vi "Pulse.vi"(0 "Data in":T1, 1 "error in":errorcluster) -> (2 "Data out":T1, 3 "error out":errorcluster, 4 "Ran?":bool)   [LabVIEW 2017, in "Steps.lvlib"]
uses:
  Steps.lvlib
  Type_Defs/Data.ctl
  Type_Defs/Diagnostics.ctl
  Type_Defs/Systems.ctl
panel:
  out "Helical":dbl(graph)
  out "Toroidal":dbl(graph)
  in  "Step Back":bool
  in  "Continue":bool
  # "Verify that the pulse is correct."
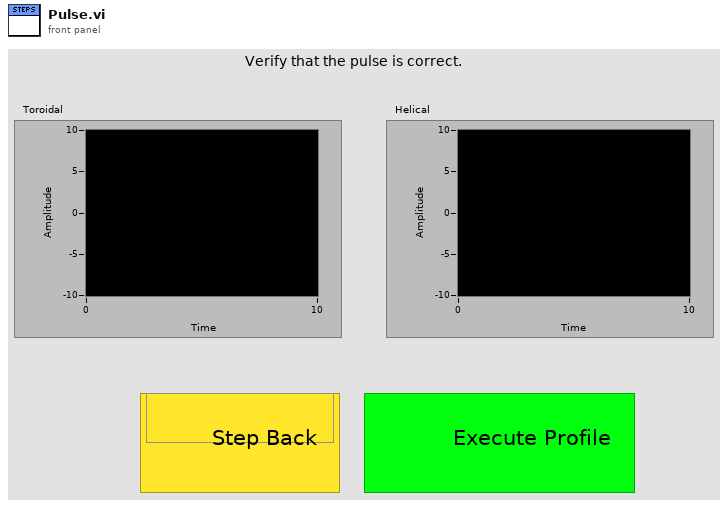
[diagram p1: front panel]
types:
  T1 = typedef "Data.ctl" = cluster{"User Name":string, "Experiment Number":i32, "Start Time":timestamp, "Data":dbl[], "Step Number":i32, "Step Instructions":string, "Diagnostics":T2, "Experiment Purpose":string, "Experiment State":enum16{"Off", "Setting Up", "Ready", "In Progress", "Shutting Down"}, "Systems":T3, "Vacuum Pressure":dbl, "Fieldpoints":cluster{"System Boolean Fieldpoints":cluster{"Compressed Air":refnum<k21>, "T-20kV Power Switch":refnum<k21>, "T-Rectifier":refnum<k21>, "Engage Interlock":refnum<k21>, "Ventilator":refnum<k21>, "Magnetron":refnum<k21>, "H-20kV Power Switch":refnum<k21>, "H-Rectifier":refnum<k21>, "Main Water Pump":refnum<k21>, "WEGA Water Pump":refnum<k21>, "Gas Inlet Valves":refnum<k21>}, "Step Fieldpoints":cluster{"Exhaust Ventillator":refnum<k21>, "Compressed Air":refnum<k21>, "Water Pressure":refnum<k21>, "Interlock":refnum<k21>, "Toroidal Power Supply 1":refnum<k21>, "Toroidal Power Supply 2":refnum<k21>, "Toroidal Rectifier":refnum<k21>, "Helical Power Supply":refnum<k21>, "Helical Rectifier":refnum<k21>, "6kW Magnetron Standby":refnum<k21>, "20kW Magnetron Standby":refnum<k21>}}, "Pressure History":cluster{"Seconds into Experiment":i32[], "Pressure Data":dbl[]}, "Time Computer Control":dbl[], "Toroidal Voltage Computer Control":dbl[], "Helical Voltage Computer Control":dbl[], "Toroidal Current":dbl[], "Toroidal Voltage":dbl[], "Toroidal Current Set Point":dbl[], "Helical Current Set Point":dbl[], "Helical Voltage":dbl[], "Helical Current":dbl[], "Experiment Folder":path, "Run Another Shot?":bool}
  T2 = typedef "Diagnostics.ctl" = cluster{"Langmuir Probe":bool, "Rogowski 1":bool, "Rogowski 2":bool, "Rogowski 3":bool, "B-dot 1":bool, "B-dot 2":bool}
  T3 = typedef "Systems.ctl" = cluster{"Compressed Air":bool, "T-20kV Power Switch":bool, "T-Rectifier":bool, "Engage Interlock":bool, "Ventilator":bool, "Magnetron":bool, "H-20kV Power Switch":bool, "H-Rectifier":bool, "Main Water Pump":bool, "WEGA Water Pump":bool, "Gas Inlet Valves":bool}
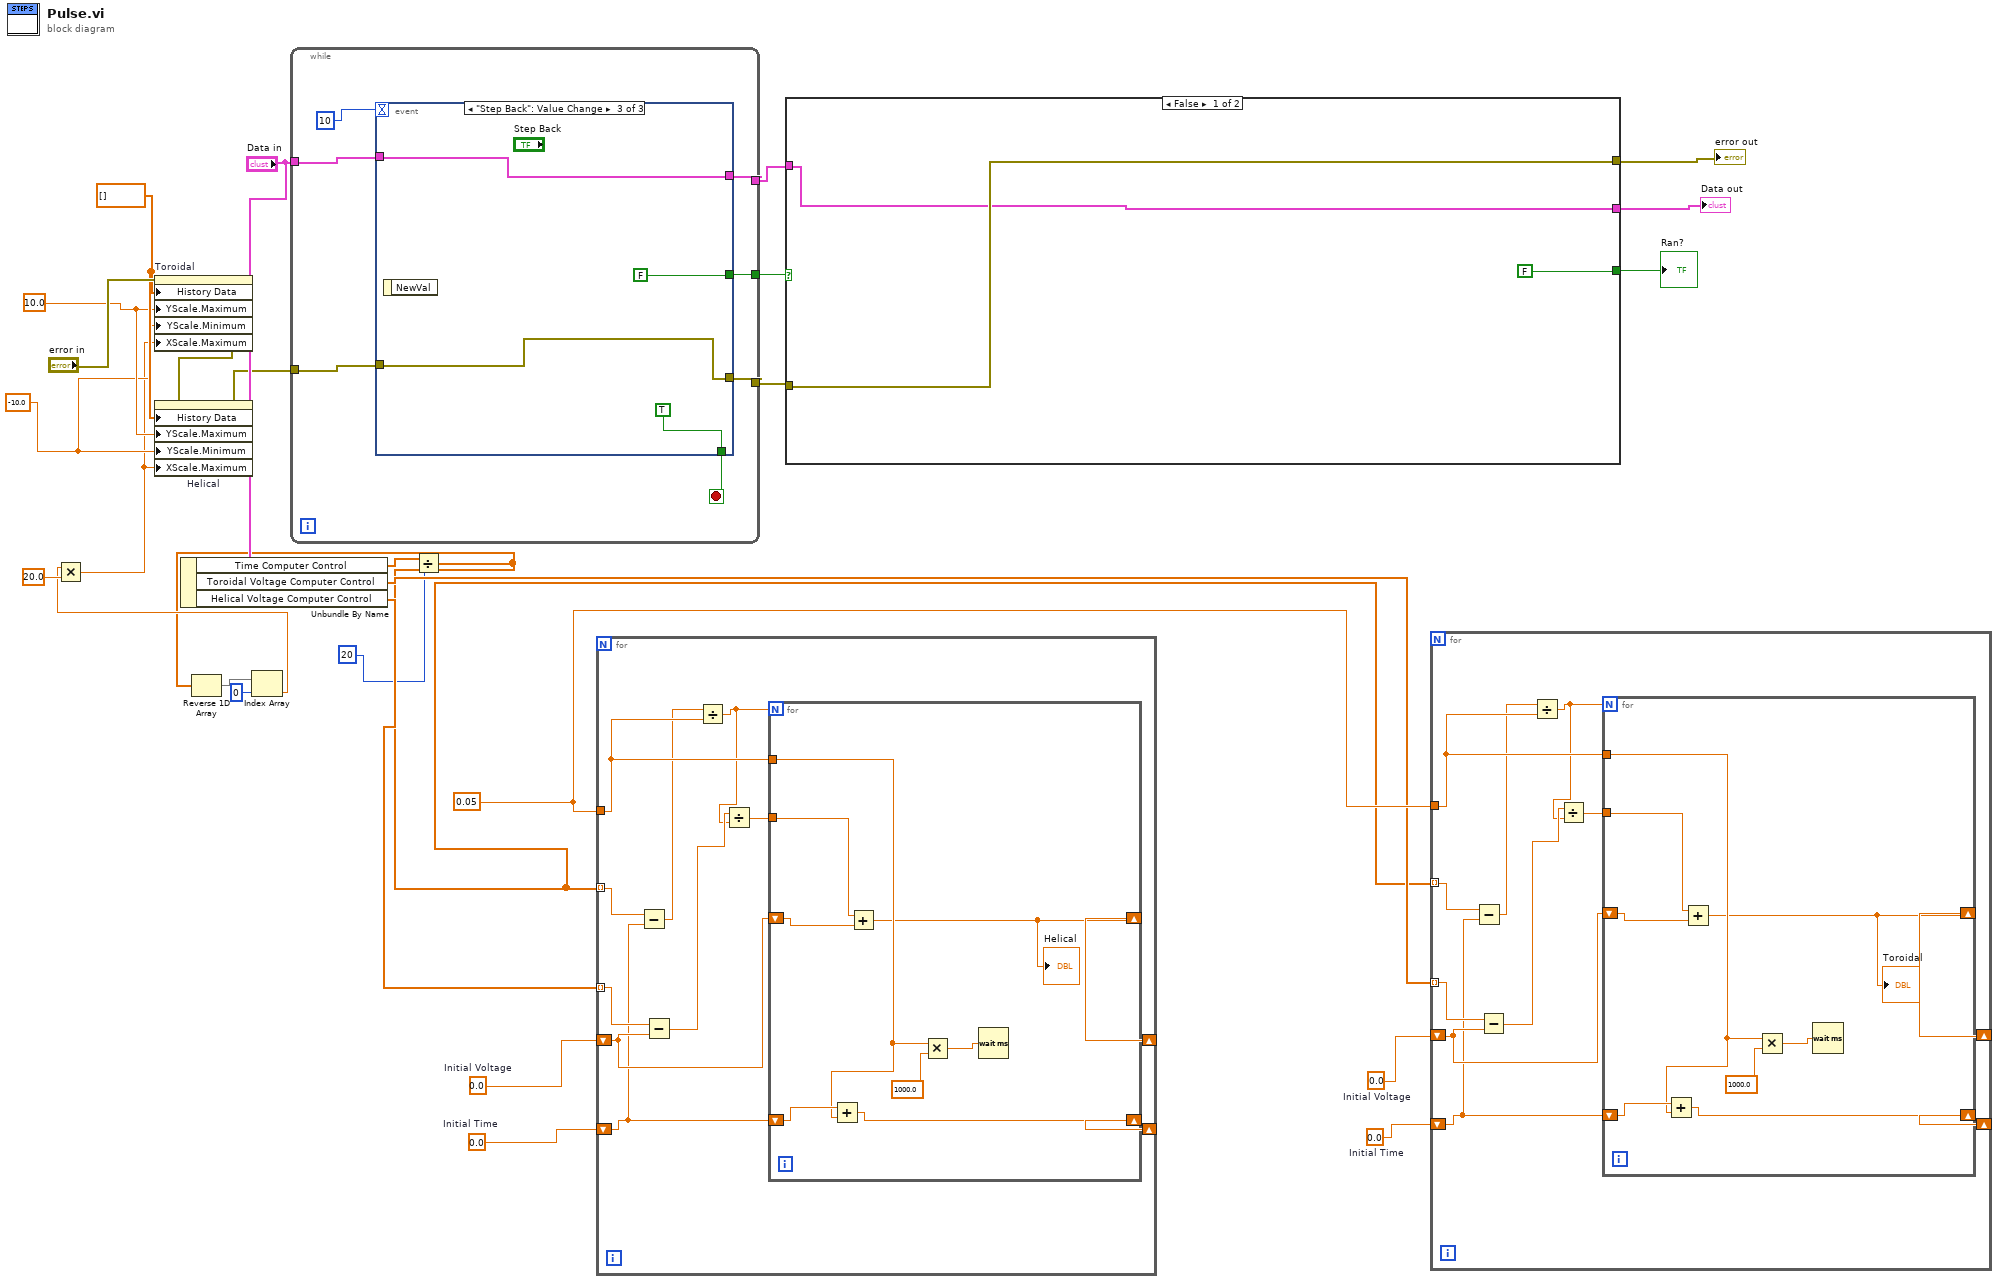
[diagram p0: block diagram]
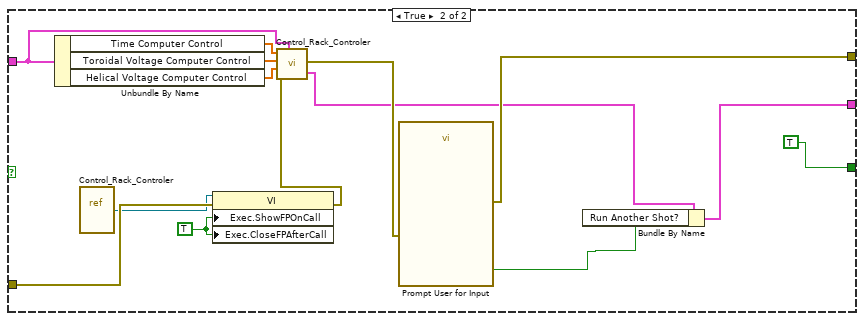
[diagram p2: hidden frame]
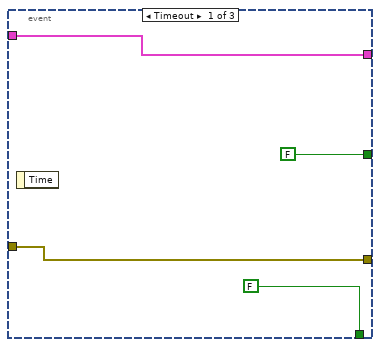
[diagram p3: hidden frame]
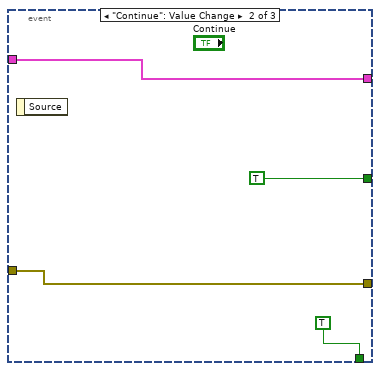
[diagram p4: hidden frame]
diagram:
  w9 = -10.0 ("Y Scale.Range:Maximum")
  w10 = 10.0 ("Y Scale.Range:Maximum")
  w13 = dbl[] [] ("History Data")
  w19 = 0.05 ("Timestep (in seconds, keep above 1/20s)")
  w21 = 0.0  # Initial Time
  w20 = 0.0  # Initial Voltage
  w22 = 0.0  # Initial Time
  w23 = 0.0  # Initial Voltage
  n1 = Unbundle By Name("Data in") -> ("Time Computer Control"=w4:dbl[], "Toroidal Voltage Computer Control"=w17:dbl[], "Helical Voltage Computer Control"=w18:dbl[])
  n2 = Divide(x=w4, y=20 ("Time Computer Control")) -> (x/y=w5:dbl[])
  n3 = Reverse 1D Array(array=w5) -> (reversed array=w12:dbl[])
  n4 = Index Array(array=w12, index=0) -> (element=w7:dbl)
  n5 = Multiply(x=w7, y=20.0) -> (x*y=w6:dbl)
  n6 = property on="Toroidal" class="WFChart (strict)"(error in="error in", "History Data"=w13, "YScale.Maximum"=w10, "YScale.Minimum"=w9, "XScale.Maximum"=w6) -> (error out=w15:errorcluster)  [unwired: 1 in, 1 out]
  n7 = property on="Helical" class="WFChart (strict)"(error in=w15, "History Data"=w13, "YScale.Maximum"=w10, "YScale.Minimum"=w9, "XScale.Maximum"=w6) -> (error out=w14:errorcluster)  [unwired: 1 in, 1 out]
  n8 = while {
    tunnel: w14 -> [w35]
    tunnel: [w34] -> w25
    tunnel: [w32] -> w27
    tunnel: "Data in" -> [w31]
    tunnel: [w29] -> w2
    stop <- w33 stop-if-true
    n9 = event shown="[2] \"Step Back\": Value Change" {
      selector: _ -> [_ _ _]
      dyn-events: _ -> [_ _ _]
      timeout: 10 -> [_ _ _]
      tunnel: w35 -> [w38 w43 w45]
      tunnel: [w38 w43 w45] -> w34
      tunnel: [FALSE TRUE TRUE] -> w33
      tunnel: [w37 w41 w46] -> w32
      tunnel: w31 -> [w37 w41 w46]
      tunnel: [FALSE TRUE FALSE] -> w29
      event Timeout {
        n10 = event-data() -> ()  [unwired: 1 in, 1 out]
      }
      event "Continue": Value Change {
        n11 = event-data() -> ()  [unwired: 1 in, 1 out]
      }
      event "Step Back": Value Change {
        n12 = event-data() -> ()  [unwired: 1 in, 1 out]
      }
    }
  }
  n13 = for {
    tunnel: w18 -> [w58] mode=indexing
    tunnel: w5 -> [w51] mode=indexing
    tunnel: w19 -> [w53]
    shift-right: [w54] -> _
    shift-left: w23 -> [w57]
    shift-right: [w52] -> _
    shift-left: w22 -> [w50]
    n14 = Subtract(x=w51, y=w50) -> (x-y=w49:dbl)
    n15 = Subtract(x=w58, y=w57) -> (x-y=w56:dbl)
    n16 = Divide(x=w49, y=w53) -> (x/y=w48:dbl)
    n17 = Divide(x=w56, y=w48) -> (x/y=w55:dbl)
    n18 = for {
      N: w48 -> [_]
      shift-right: [w59] -> w54
      shift-left: w57 -> [w66]
      tunnel: w55 -> [w65]
      tunnel: w53 -> [w62]
      shift-right: [w60] -> w52
      shift-left: w50 -> [w64]
      n19 = Add(x=w64, y=w62) -> (x+y=w60:dbl)
      n20 = Add(x=w65, y=w66) -> (x+y=w59:dbl)
      "Helical" <- w59
      n21 = Multiply(x=w62, y=1000.0) -> (x*y=w63:dbl)
      n22 = Wait (ms)(milliseconds to wait=w63) -> ()  [unwired: 1 out]
    }
  }
  n23 = case shown="False" w2 {
    tunnel: [w69 w73] -> w28
    tunnel: w27 -> [w68 w80]
    tunnel: [w68 w71] -> w26
    tunnel: w25 -> [w69 w78]
    tunnel: [FALSE TRUE] -> w1
    frame False {
    }
    frame True {
      w79 = TRUE ("Execution:Show Front Panel On Call")
      n24 = Unbundle By Name(w80) -> ("Time Computer Control"=w83:dbl[], "Toroidal Voltage Computer Control"=w82:dbl[], "Helical Voltage Computer Control"=w81:dbl[])
      n25 = vi-ref "Control_Rack_Controler.vi"() -> (w76:refnum<vi>)
      n26 = property class="VI"(reference=w76, error in=w78, "Exec.ShowFPOnCall"=w79, "Exec.CloseFPAfterCall"=w79) -> (error out=w77:errorcluster)  [unwired: 1 out]
      n27 = call "Control_Rack_Controler.vi"("Times"=w83, "Voltages Toroidal (Keep below |10|)"=w82, "Voltages Helical (Keep below |10|)"=w81, "error out"=w77, "Data out 2"=w80) -> ("error out 2"=w74:errorcluster, "Data out"=w72:T1)
      n28 = call "Prompt User for Input"("error in (no error)"=w74) -> ("Run New Shot"=w75:bool, "error out"=w73:errorcluster)  [unwired: 16 in, 1 out]
      n29 = Bundle By Name(cluster=w72, "Run Another Shot?"=w75) -> (w71:T1)
    }
  }
  "error out" <- w28
  "Data out" <- w26
  "Ran?" <- w1
  n30 = for {
    tunnel: w17 -> [w94] mode=indexing
    tunnel: w5 -> [w87] mode=indexing
    tunnel: w19 -> [w89]
    shift-right: [w90] -> _
    shift-left: w20 -> [w93]
    shift-right: [w88] -> _
    shift-left: w21 -> [w86]
    n31 = Subtract(x=w87, y=w86) -> (x-y=w85:dbl)
    n32 = Subtract(x=w94, y=w93) -> (x-y=w92:dbl)
    n33 = Divide(x=w85, y=w89) -> (x/y=w84:dbl)
    n34 = Divide(x=w92, y=w84) -> (x/y=w91:dbl)
    n35 = for {
      N: w84 -> [_]
      shift-right: [w95] -> w90
      shift-left: w93 -> [w102]
      tunnel: w91 -> [w101]
      tunnel: w89 -> [w98]
      shift-right: [w96] -> w88
      shift-left: w86 -> [w100]
      n36 = Add(x=w100, y=w98) -> (x+y=w96:dbl)
      n37 = Add(x=w101, y=w102) -> (x+y=w95:dbl)
      "Toroidal" <- w95
      n38 = Multiply(x=w98, y=1000.0) -> (x*y=w99:dbl)
      n39 = Wait (ms)(milliseconds to wait=w99) -> ()  [unwired: 1 out]
    }
  }
